vi "Get Next Actor.vi"(8 "error in (no error)":errorcluster, 11 "Pipelined Actor in":refnum<class "Pipelined Actor.lvclass">) -> (0 "error out":errorcluster, 2 "Message Enqueuer":refnum<class "Message Enqueuer.lvclass">, 3 "Pipelined Actor out":refnum<class "Pipelined Actor.lvclass">)   [LabVIEW 2014, in "Pipelined Actor.lvlib" / "Pipelined Actor.lvclass"]
uses:
  Pipelined Actor.lvclass
  <vilib>/ActorFramework/Message Enqueuer/Message Enqueuer.lvclass
  Pipelined Actor.lvclass/Pipelined Actor.ctl
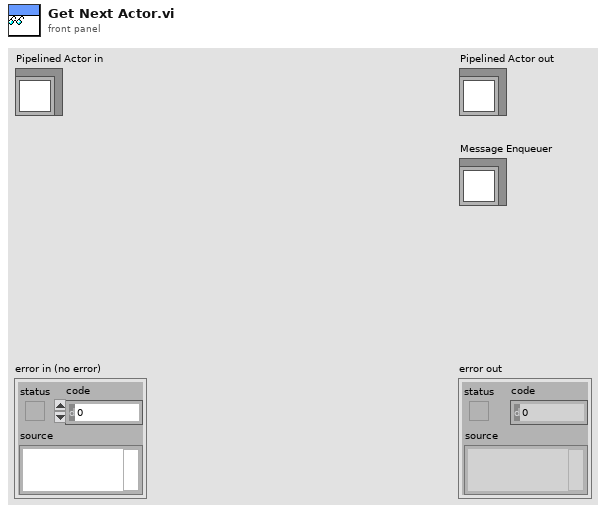
[diagram p1: front panel]
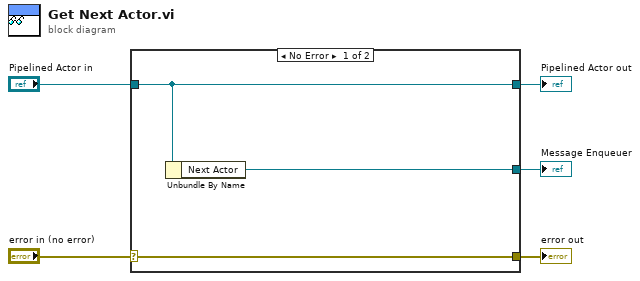
[diagram p0: block diagram]
diagram:
  n1 = case shown="No Error" "error in (no error)" {
    selector: "error in (no error)" -> [w8 w9]
    tunnel: [w8 w9] -> w4
    tunnel: [w7 w10] -> w2
    tunnel: "Pipelined Actor in" -> [w7 w10]
    tunnel: [w6 _] -> w1
    frame No Error {
      n2 = Unbundle By Name(w7) -> ("Next Actor"=w6:refnum<class "Message Enqueuer.lvclass">)
    }
    frame Error {
    }
  }
  "error out" <- w4
  "Pipelined Actor out" <- w2
  "Message Enqueuer" <- w1
